vi "Update Splash.vi"(8 "error in (no error)":errorcluster, 10 "Status":string, 11 "Splash Screen in":refnum<class "Splash Screen.lvclass">) -> (0 "error out":errorcluster, 3 "Splash Screen out":refnum<class "Splash Screen.lvclass">)   [LabVIEW 2020, in "Volatus.lvlib" / "Splash Screen.lvclass"]
uses:
  Splash Screen.lvclass
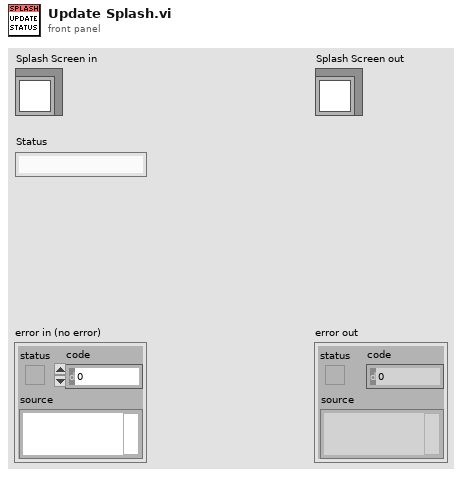
[diagram p1: front panel]
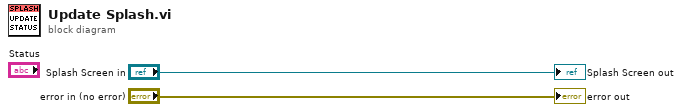
[diagram p0: block diagram]
diagram:
  "error out" <- "error in (no error)"
  "Splash Screen out" <- "Splash Screen in"
